vi "texture fault detect.vi"() -> ()   [LabVIEW 2021]
uses:
  <vilib>/vision/Classification.llb/IMAQ SVM Kernel Options.ctl
  <vilib>/vision/Classification.llb/IMAQ SVM Model Options.ctl
  <vilib>/vision/Classification.llb/IMAQ Classifier Read Options.ctl
  37daa565-0501-4398-9aa0-111dd2159123.vi
  <vilib>/vision/NI_Vision_Development_Module.lvlib
panel:
  in  "Min. Defect Identification Score":dbl=600.0
  out "number of fault":i32
  out "Image":T1(plugin-control)
  in  "Model Options":T2={"SVM Model"=enum."One Class", "Tolerance"=0.001, "Max. Iteration"=100000, "Nu"=0.1, "Shrinking"=TRUE, "Cost"=1.0, "Weighted Cost"=[]}
  in  "Kernel Options":T3={"Kernel"=enum."RBF", "Degree"=3, "Gamma"=1.0, "Coefficient"=0.0, "Sigma"=1.0, "Cache(MB)"=10.0}
  in  "Co-occurrence Options":T4={"  Level"=16, "Displacement Vector"={"xDelta"=1, "yDelta"=1}} {"Displacement Vector"."yDelta" min=1 step=1; "Displacement Vector"."xDelta" min=1 step=1}
  in  "Window Options":T5={"SizeX"=32, "SizeY"=32, "Step Size"=0}
  in  "Wavelet Options":T6={"Type"=14, "Wavelet Banks To Use"=[0, 1, 2, 3, 4, 5, 6, 7], "Min. Energy Level"=100.0} {"Min. Energy Level" min=0 max=100; "Wavelet Banks To Use" items=["Low Low", "Low High", "High Low", "High High", "Low Low Low", "Low Low High", "Low High Low", "Low High High"]; "Type" items=["db02"=0, "db03"=1, "db04"=2, "db05"=3, "db06"=4, "db07"=5, "db08"=6, "db09"=7, "db10"=8, "db11"=9, "db12"=10, "db13"=11, "db14"=12, "Haar"=13, "bior1_3"=14, "bior1_5"=15, "bior2_2"=16, "bior2_4"=17, "bior2_6"=18, "bior2_8"=19, "bior3_1"=20, "bior3_3"=21, "bior3_5"=22, "bior3_7"=23, "bior3_9"=24, "bior4_4 (FBI)"=25, "bior5_5"=38, "bior6_8"=39, "coif1"=26, "coif2"=27, "coif3"=28, "coif4"=29, "coif5"=30, "sym2"=31, "sym3"=32, "sym4"=33, "sym5"=34, "sym6"=35, "sym7"=36, "sym8"=37]}
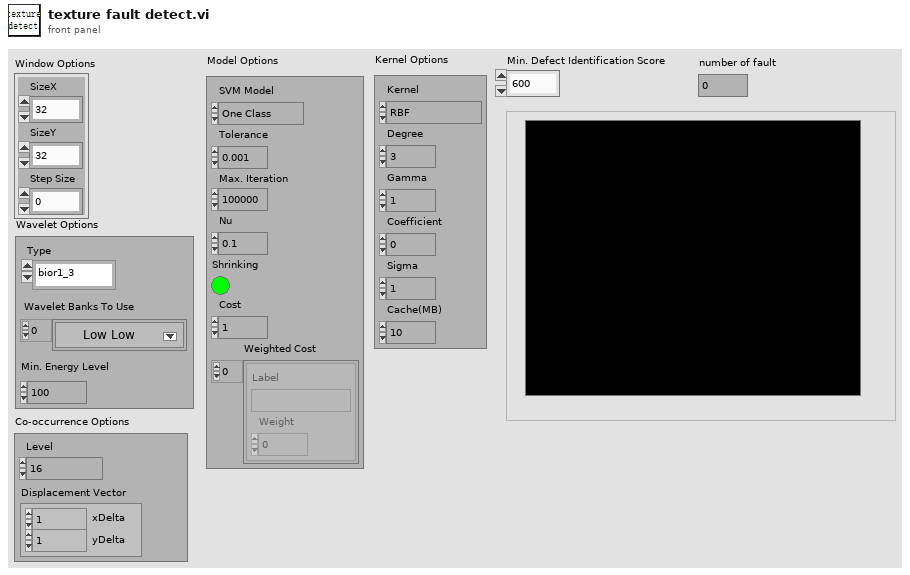
[diagram p1: front panel]
types:
  T1 = typedef "IMAQ Image.ctl" = refnum<image>
  T2 = typedef "IMAQ SVM Model Options.ctl" = cluster{"SVM Model":enum32{"C-SVC", "nu-SVC", "One Class"}, "Tolerance":dbl, "Max. Iteration":i32, "Nu":dbl, "Shrinking":bool, "Cost":dbl, "Weighted Cost":cluster{"Label":string, "Weight":dbl}[]}
  T3 = typedef "IMAQ SVM Kernel Options.ctl" = cluster{"Kernel":enum32{"Linear", "Polynomial", "Gaussian", "RBF"}, "Degree":i32, "Gamma":dbl, "Coefficient":dbl, "Sigma":dbl, "Cache(MB)":dbl}
  T4 = cluster{"  Level":i32, "Displacement Vector":cluster{"xDelta":i32, "yDelta":i32}}
  T5 = cluster{"SizeX":i32, "SizeY":i32, "Step Size":i32}
  T6 = cluster{"Type":i32, "Wavelet Banks To Use":i32[], "Min. Energy Level":sgl}
  T7 = typedef "IMAQ Classifier Read Options.ctl" = i32
  T8 = typedef "Image Type" = u32
  T9 = typedef "IMAQ Classifier Session.ctl" = refnum<k1>
  T10 = typedef "ROI Descriptor" = cluster{"Global Rectangle":i32[], "Contours":cluster{"ID":enum32{"External", "Internal"}, "Type":u32, "Coordinates":i32[]}[]}
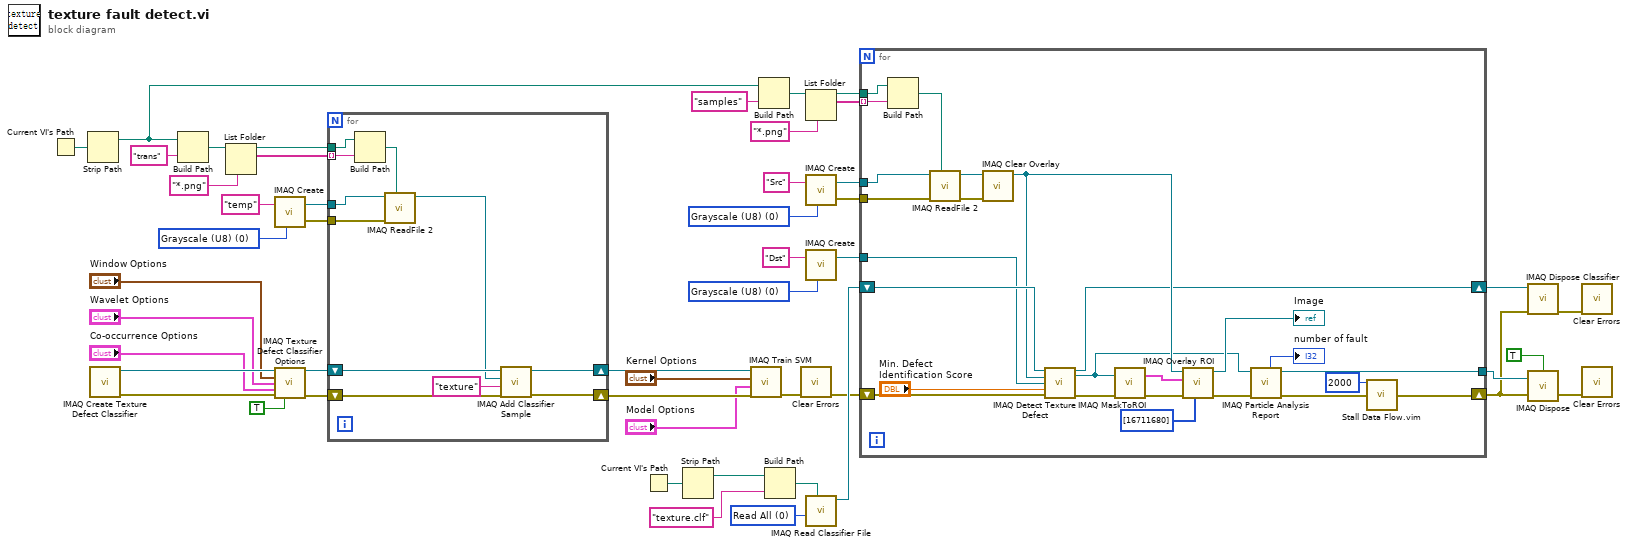
[diagram p0: block diagram]
diagram:
  w1 = T7 0 items=["Read All", "Add Samples, Do Not Change Options", "Read Options, Do Not Add Samples"] ("Read Options")
  w6 = T8 0 items=["Grayscale (U8)", "Grayscale (I16)", "Grayscale (SGL)", "Complex (CSG)", "RGB (U32)", "HSL (U32)", "RGB (U64)", "Grayscale (U16)"] ("Image Type")
  w5 = T8 0 items=["Grayscale (U8)", "Grayscale (I16)", "Grayscale (SGL)", "Complex (CSG)", "RGB (U32)", "HSL (U32)", "RGB (U64)", "Grayscale (U16)"] ("Image Type")
  w45 = T8 0 items=["Grayscale (U8)", "Grayscale (I16)", "Grayscale (SGL)", "Complex (CSG)", "RGB (U32)", "HSL (U32)", "RGB (U64)", "Grayscale (U16)"] ("Image Type")
  n1 = Current VI's Path() -> (path=w49:path)
  n2 = Strip Path(path=w49) -> (stripped path=w26:path)  [unwired: 1 out]
  n3 = call "IMAQ Create Texture Defect Classifier"() -> ("error out"=w40:errorcluster, "Classifier Session Out"=w41:T9)  [unwired: 10 in]
  n4 = Build Path(base path=w26, name or relative path="trans") -> (appended path=w29:path)
  n5 = List Folder(path=w29, pattern="*.png" ("类型")) -> (path out=w46:path, filenames=w47:string[])  [unwired: 2 in, 2 out]
  n6 = call "IMAQ Create"("Image Name"="temp", "Image Type"=w45) -> ("New Image"=w43:T1, "error out"=w42:errorcluster)  [unwired: 3 in]
  n7 = call "IMAQ Texture Defect Classifier Options"("Classifier Session"=w41, "Window Options"="Window Options", "Wavelet Options"="Wavelet Options", "Co-occurrence Options"="Co-occurrence Options", "error in (no error)"=w40, "Get/Set Options? (Get)"=TRUE) -> ("Classifier Session (dup)"=w36:T9, "error out"=w35:errorcluster)  [unwired: 5 in, 3 out]
  n8 = for {
    tunnel: w47 -> [w60] mode=indexing
    tunnel: w46 -> [w59]
    tunnel: w43 -> [w57]
    tunnel: w42 -> [w56]
    shift-right: [w52] -> w33
    shift-left: w36 -> [w55]
    shift-right: [w51] -> w32
    shift-left: w35 -> [w54]
    n9 = Build Path(base path=w59, name or relative path=w60) -> (appended path=w58:path)
    n10 = call "IMAQ ReadFile 2"("File Path"=w58, "error in (no error)"=w56, "Image"=w57) -> ("Image Out"=w50:T1)  [unwired: 4 in, 4 out]
    n11 = call "IMAQ Add Classifier Sample"("error in (no error)"=w54, "Class"="texture", "Image"=w50, "Classifier Session"=w55) -> ("error out"=w51:errorcluster, "Classifier Session (dup)"=w52:T9)  [unwired: 5 in, 1 out]
  }
  n12 = Current VI's Path() -> (path=w13:path)
  n13 = Strip Path(path=w13) -> (stripped path=w12:path)  [unwired: 1 out]
  n14 = call "IMAQ Train SVM"("error in (no error)"=w32, "Model Options"="Model Options", "Kernel Options"="Kernel Options", "Classifier Session"=w33) -> ("error out"=w4:errorcluster)  [unwired: 4 in, 3 out]
  n15 = Build Path(base path=w26, name or relative path="samples") -> (appended path=w24:path)
  n16 = Build Path(base path=w12, name or relative path="texture.clf") -> (appended path=w11:path)
  n17 = call <vilib>:"Clear Errors.vi"("error in (no error)"=w4) -> ("error out"=w3:errorcluster)  [unwired: 5 in, 1 out]
  n18 = List Folder(path=w24, pattern="*.png" ("类型")) -> (path out=w23:path, filenames=w22:string[])  [unwired: 2 in, 2 out]
  n19 = call "IMAQ Create"("Image Name"="Src", "Image Type"=w5) -> ("New Image"=w20:T1, "error out"=w19:errorcluster)  [unwired: 3 in]
  n20 = call "IMAQ Create"("Image Name"="Dst", "Image Type"=w6) -> ("New Image"=w18:T1)  [unwired: 3 in, 1 out]
  n21 = call "IMAQ Read Classifier File"("File Path"=w11, "Read Options"=w1) -> ("Classifier Session"=w10:T9)  [unwired: 5 in, 4 out]
  n22 = for {
    tunnel: w23 -> [w85]
    tunnel: w22 -> [w67] mode=indexing
    tunnel: w20 -> [w62]
    tunnel: w19 -> [w66]
    tunnel: w18 -> [w82]
    shift-right: [w70] -> w8
    shift-left: w3 -> [w83]
    tunnel: [w72] -> w16
    shift-right: [w68] -> w9
    shift-left: w10 -> [w84]
    n23 = Build Path(base path=w85, name or relative path=w67) -> (appended path=w63:path)
    n24 = call "IMAQ ReadFile 2"("File Path"=w63, "error in (no error)"=w66, "Image"=w62) -> ("error out"=w65:errorcluster, "Image Out"=w64:T1)  [unwired: 4 in, 3 out]
    n25 = call "IMAQ Clear Overlay"("error in (no error)"=w65, "Image"=w64) -> ("Image Out"=w79:T1)  [unwired: 1 in, 8 out]
    n26 = call "IMAQ Detect Texture Defect"("Classifier Session"=w84, "Image Src"=w79, "Image Dst"=w82, "Min. Defect Identification Score"="Min. Defect Identification Score", "error in (no error)"=w83) -> ("Classifier Session (dup)"=w68:T9, "Image Dst Out"=w74:T1, "error out"=w81:errorcluster)  [unwired: 8 in]
    n27 = call "IMAQ MaskToROI"("Image"=w74, "error in (no error)"=w81) -> ("ROI Descriptor"=w78:T10, "error out"=w80:errorcluster)  [unwired: 5 in, 1 out]
    n28 = call "IMAQ Overlay ROI"("Colors (Green)"=u32[] [16711680], "error in (no error)"=w80, "ROI Descriptor"=w78, "Image"=w79) -> ("error out"=w76:errorcluster, "Image Out"=→"Image":T1)  [unwired: 6 in]
    n29 = call "IMAQ Particle Analysis Report"("error in (no error)"=w76, "Image"=w74) -> ("error out"=w71:errorcluster, "Image Out (duplicate)"=w72:T1, "Number of Particles"=→"number of fault":i32)  [unwired: 4 in, 3 out]
    n30 = call "Stall Data Flow.vim"("value in"=w71, "milliseconds to wait"=u32 2000) -> ("value out"=w70:errorcluster)  [unwired: 1 out]
  }
  n31 = call "IMAQ Dispose Classifier"("error in (no error)"=w8, "Classifier Session"=w9) -> ("error out"=w7:errorcluster)  [unwired: 9 in]
  n32 = call "IMAQ Dispose"("All Images? (No)"=TRUE, "Image"=w16, "error in (no error)"=w8) -> ("error out"=w14:errorcluster)  [unwired: 3 in]
  n33 = call <vilib>:"Clear Errors.vi"("error in (no error)"=w7) -> ()  [unwired: 5 in, 2 out]
  n34 = call <vilib>:"Clear Errors.vi"("error in (no error)"=w14) -> ()  [unwired: 5 in, 2 out]
